vi "PumpController GetSensorReading.vi"(6 "contextId":T1, 8 "error in":errorcluster, 9 "timeout (ms)":i32=-1, 10 "Request Data":T3, 11 "gRPC ID":T1) -> (0 "error out":errorcluster, 2 "Response Data":T2, 3 "gRPC ID out":T1)   [LabVIEW 2024, in "pumploop_client.lvlib"]
uses:
  pumploop_client.lvlib
  <vilib>/gRPC/LabVIEW gRPC Library/Shared/grpcId.ctl
  RPC Messages/pumploop_GetSensorRequest.ctl
  RPC Messages/pumploop_Sensors.ctl
  RPC Messages/pumploop_Sensors_Flat.ctl
  14035477-4c25-4107-8ed5-d0c4ef420ce5.vi
  <vilib>/gRPC/LabVIEW gRPC Library/Shared/TranslateGrpcError.vi
  <vilib>/gRPC/LabVIEW gRPC Library/Server API/Server/Get Server DLL Path.vi
  <vilib>/Utility/error.llb/Error Cluster From Error Code.vi
  <vilib>/gRPC/LabVIEW gRPC Library/Shared/Wait On Occurrence Wrapper.vi
  <vilib>/gRPC/LabVIEW gRPC Library/grpc-lvsupport-release.lvlib
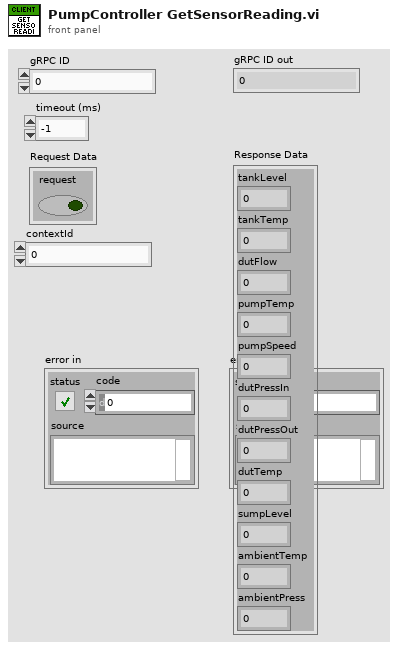
[diagram p1: front panel]
types:
  T1 = typedef "grpc-lvsupport-release.lvlib/grpcId.ctl" = u64
  T2 = typedef "pumploop_client.lvlib/pumploop_Sensors.ctl" = cluster{"tankLevel":sgl, "tankTemp":sgl, "dutFlow":sgl, "pumpTemp":sgl, "pumpSpeed":sgl, "dutPressIn":sgl, "dutPressOut":sgl, "dutTemp":sgl, "sumpLevel":sgl, "ambientTemp":sgl, "ambientPress":sgl}
  T3 = typedef "pumploop_client.lvlib/pumploop_GetSensorRequest.ctl" = cluster{"request":bool}
  T4 = typedef "pumploop_client.lvlib/pumploop_Sensors_Flat.ctl" = cluster{"tankLevel":sgl, "tankTemp":sgl, "dutFlow":sgl, "pumpTemp":sgl, "pumpSpeed":sgl, "dutPressIn":sgl, "dutPressOut":sgl, "dutTemp":sgl, "sumpLevel":sgl, "ambientTemp":sgl, "ambientPress":sgl}
  T5 = typedef "pumploop_client.lvlib/pumploop_GetSensorRequest_Flat.ctl" = cluster{"request":bool}
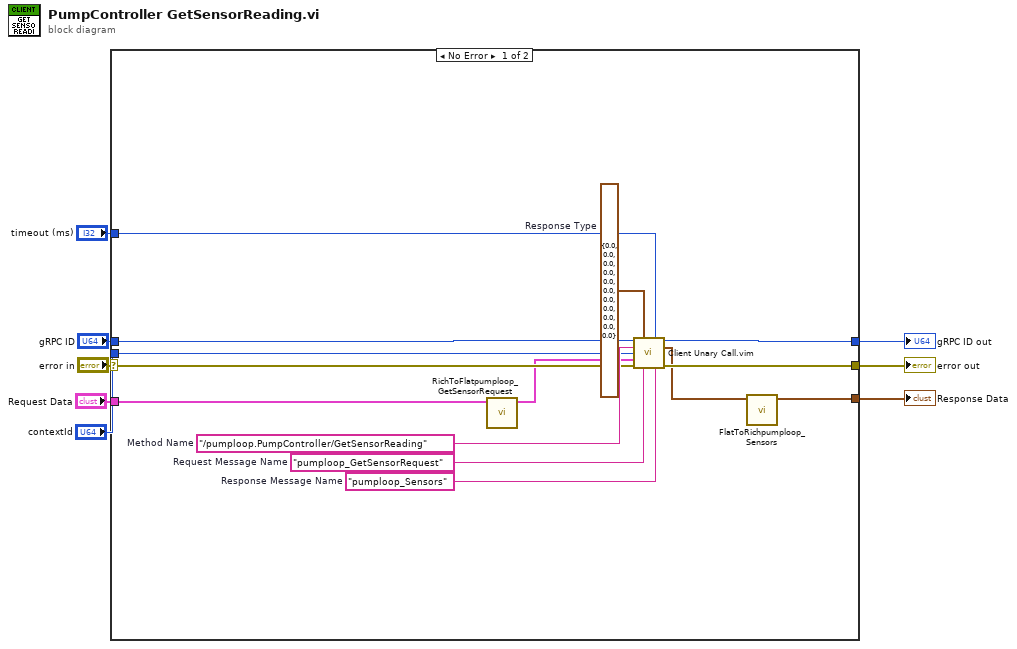
[diagram p0: block diagram]
diagram:
  n1 = case shown="No Error" "error in" {
    selector: "error in" -> [w18 w23]
    tunnel: [w17 w23] -> w7
    tunnel: "gRPC ID" -> [w16 w24]
    tunnel: [w15 w24] -> w5
    tunnel: "Request Data" -> [w12 _]
    tunnel: [w9 _] -> w3
    tunnel: "timeout (ms)" -> [w14 _]
    tunnel: "contextId" -> [w13 _]
    frame No Error {
      w19 = "pumploop_Sensors"  # Response Message Name
      w20 = "pumploop_GetSensorRequest"  # Request Message Name
      w21 = T4 {"tankLevel"=0.0, "tankTemp"=0.0, "dutFlow"=0.0, "pumpTemp"=0.0, "pumpSpeed"=0.0, "dutPressIn"=0.0, "dutPressOut"=0.0, "dutTemp"=0.0, "sumpLevel"=0.0, "ambientTemp"=0.0, "ambientPress"=0.0}  # Response Type
      w22 = "/pumploop.PumpController/GetSensorReading"  # Method Name
      n2 = call "RichToFlatpumploop_GetSensorRequest.vi"("InputCluster"=w12) -> ("OutputCluster"=w11:T5)  [unwired: 10 in]
      n3 = call "Client Unary Call.vim"("ClientID in"=w16, "Response Type"=w21, "timeout (ms)"=w14, "Method Name"=w22, "contextId"=w13, "Request Data"=w11, "error in"=w18, "Request Message Name"=w20, "Response Message Name"=w19) -> ("ClientID out"=w15:u64, "Response Data"=w10:T4, "error out"=w17:errorcluster)  [unwired: 4 in]
      n4 = call "FlatToRichpumploop_Sensors.vi"("InputCluster"=w10) -> ("OutputCluster"=w9:T2)  [unwired: 10 in]
    }
    frame Error {
    }
  }
  "error out" <- w7
  "gRPC ID out" <- w5
  "Response Data" <- w3
